vi "ExitReminder.vi"(1 "message":string) -> (0 "Exit":bool)   [LabVIEW 2015]
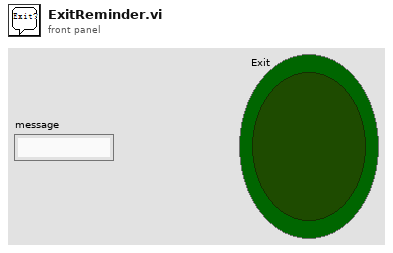
[diagram p1: front panel]
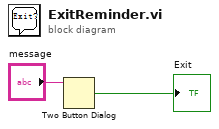
[diagram p0: block diagram]
diagram:
  n1 = Two Button Dialog(message="message") -> (T button?=→"Exit":bool)  [unwired: 2 in]
